vi "Compute Tag Angles.vi"(4 "Angle Mode":enum16{"Barrel View", "360 View"}(ring), 6 "Split Image Info":T4={"height"=120.0, "width"=120.0, "deg/pix"=120.0}, 9 "IMU offset":dbl, 10 "tag info":dbl[][](array[numeric]), 11 "Detections":T1[](array[typedef])) -> (2 "Vectors":cluster{cluster{"X":dbl, "Y":dbl}[]}[](array[cluster]), 3 "updated tags":T5(array[cluster]))   [LabVIEW 2025]
uses:
  <vilib>/Serenial/G Augmented-Reality Toolkit/g_ar_toolkit.feature_detection/Apriltag Detector/Detection.ctl
  <vilib>/Serenial/G Augmented-Reality Toolkit/g_ar_toolkit.common/Image Point (Float).ctl
  <vilib>/Serenial/G Augmented-Reality Toolkit/g_ar_toolkit.common/Quad Corners.ctl
  <vilib>/Serenial/G Augmented-Reality Toolkit/g_ar_toolkit.common/g_ar_toolkit.common.lvlib
  <vilib>/Serenial/G Augmented-Reality Toolkit/g_ar_toolkit.feature_detection/Apriltag Detector/AprilTag Detector.lvclass
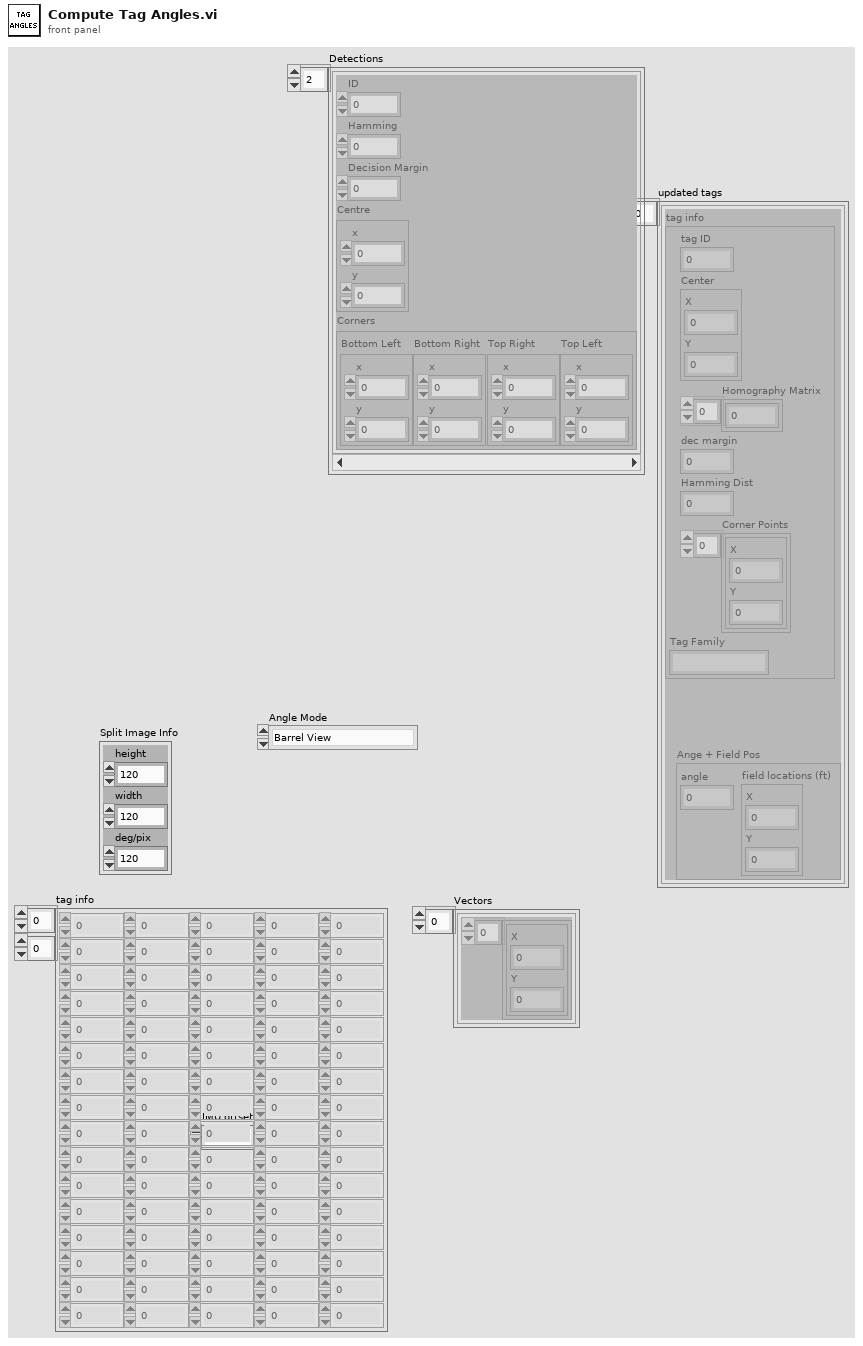
[diagram p1: front panel]
types:
  T1 = typedef "g_ar_toolkit.feature_detection.lvlib/AprilTag Detector.lvclass/Detection.ctl" = cluster{"ID":i32, "Hamming":i32, "Decision Margin":sgl, "Centre":T2, "Corners":T3}
  T2 = typedef "g_ar_toolkit.common.lvlib/Image Point (Float).ctl" = cluster{"x":dbl, "y":dbl}
  T3 = typedef "g_ar_toolkit.common.lvlib/Quad Corners.ctl" = cluster{"Bottom Left":T2, "Bottom Right":T2, "Top Right":T2, "Top Left":T2}
  T4 = cluster{"height":dbl, "width":dbl, "deg/pix":dbl}
  T5 = cluster{"tag info":cluster{"tag ID":i32, "Center":cluster{"X":dbl, "Y":dbl}, "Homography Matrix":dbl[], "dec margin":dbl, "Hamming Dist":i32, "Corner Points":cluster{"X":dbl, "Y":dbl}[], "Tag Family":string}, "Ange + Field Pos":cluster{"angle":dbl, "field locations (ft)":cluster{"X":dbl, "Y":dbl}}}[]
  T6 = cluster{"tag ID":i32, "Center":cluster{"X":dbl, "Y":dbl}, "Homography Matrix":dbl[], "dec margin":dbl, "Hamming Dist":i32, "Corner Points":cluster{"X":dbl, "Y":dbl}[], "Tag Family":string}
  T7 = cluster{"angle":dbl, "field locations (ft)":cluster{"X":dbl, "Y":dbl}}
  T8 = cluster{"tag info":cluster{"tag ID":i32, "Center":cluster{"X":dbl, "Y":dbl}, "Homography Matrix":dbl[], "dec margin":dbl, "Hamming Dist":i32, "Corner Points":cluster{"X":dbl, "Y":dbl}[], "Tag Family":string}, "Angle + Field Locations":cluster{"angle":dbl, "field locations (ft)":cluster{"X":dbl, "Y":dbl}}}
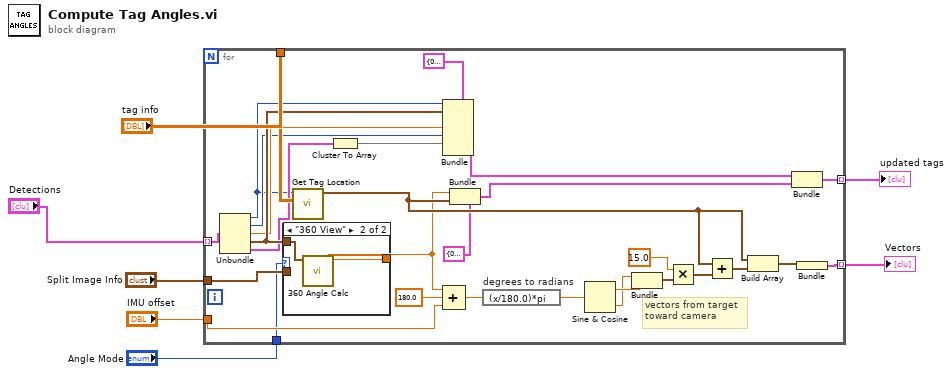
[diagram p0: block diagram]
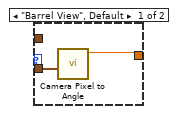
[diagram p2: hidden frame]
diagram:
  n1 = for {
    tunnel: "tag info" -> [w36]
    tunnel: [w34] -> w6 mode=indexing
    tunnel: [w23] -> w5 mode=indexing
    tunnel: "IMU offset" -> [w22]
    tunnel: "Split Image Info" -> [w20]
    tunnel: "Angle Mode" -> [w18]
    tunnel: "Detections" -> [w16] mode=indexing
    # "vectors from target\ntoward camera"
    n2 = Unbundle(w16) -> ("ID"=w8:i32, "Hamming"=w12:i32, "Decision Margin"=w13:sgl, "Centre"=w15:T2, "Corners"=w10:T3)
    n3 = case shown="\"360 View\"" w18 {
      tunnel: w20 -> [w38 _]
      tunnel: [w37 w40] -> w19
      tunnel: w15 -> [_ w39]
      frame "Barrel View", Default {
        n4 = call "Camera Pixel to Angle.vi"("Split Image Info"=w38) -> ("angle"=w37:dbl)  [unwired: 10 in]
      }
      frame "360 View" {
        n5 = call "360 Angle Calc.vi"("Center"=w39) -> ("angle"=w40:dbl)  [unwired: 10 in]
      }
    }
    n6 = call "Get Tag Location.vi"("tag info"=w36, "tag ID"=w8) -> ("field locations (ft)"=w21:cluster{"X":dbl, "Y":dbl})  [unwired: 8 in, 1 out]
    n7 = Cluster To Array(cluster=w10) -> (array=w11:T2[])
    n8 = Bundle(cluster=T6 {"tag ID"=0, "Center"={"X"=0.0, "Y"=0.0}, "Homography Matrix"=[], "dec margin"=0.0, "Hamming Dist"=0, "Corner Points"=[], "Tag Family"=""} ("tag info"), "tag ID"=w8, "Center"=w15, "dec margin"=w13, "Hamming Dist"=w12, "Corner Points"=w11) -> (w9:T6)  [unwired: 2 in]
    n9 = Compound Arithmetic op=ADD(w19, 180.0 ("y"), w22) -> (w32:dbl)
    n10 = Bundle(cluster=T7 {"angle"=0.0, "field locations (ft)"={"X"=0.0, "Y"=0.0}} ("Angle + Field Locations"), "angle"=w19, "field locations (ft)"=w21) -> (w35:T7)
    n11 = expression code="(x/180.0)*pi" "degrees to radians"(w32) -> (w31:dbl)
    n12 = Sine & Cosine(0:w31) -> (1:w30:dbl, 2:w29:dbl)
    n13 = Bundle(w29, w30) -> (w28:cluster{dbl, dbl})  [unwired: 1 in]
    n14 = Multiply(x=15.0, y=w28) -> (x*y=w27:cluster{dbl, dbl})
    n15 = Add(x=w21, y=w27) -> (x+y=w25:cluster{dbl, dbl})
    n16 = Build Array(w21, w25) -> (w24:cluster{"X":dbl, "Y":dbl}[])
    n17 = Bundle("tag info"=w9, "Angle + Field Locations"=w35) -> (w34:T8)  [unwired: 1 in]
    n18 = Bundle(w24) -> (w23:cluster{cluster{"X":dbl, "Y":dbl}[]})  [unwired: 1 in]
  }
  "updated tags" <- w6
  "Vectors" <- w5
